vi "Save.vi"(8 "error in (no error)":errorcluster, 10 "Control path":path, 11 "ctl in":refnum<class "ctl.lvclass">) -> (0 "error out":errorcluster, 3 "ctl out":refnum<class "ctl.lvclass">)   [LabVIEW 2012, in "ctl.lvclass"]
uses:
  ctl.lvclass
  ctl.lvclass/ctl.ctl
  _ResManager_v86/IDCloneResMgr.lvlib
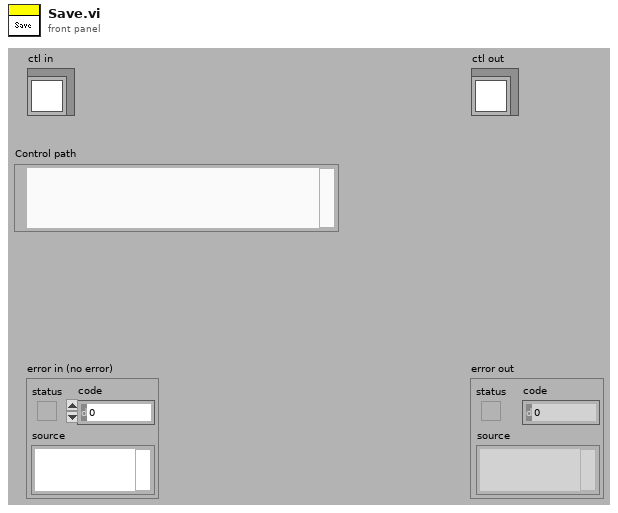
[diagram p1: front panel]
types:
  T1 = cluster{"type":u32, "id":i32, "name":string, "binary data":string}[]
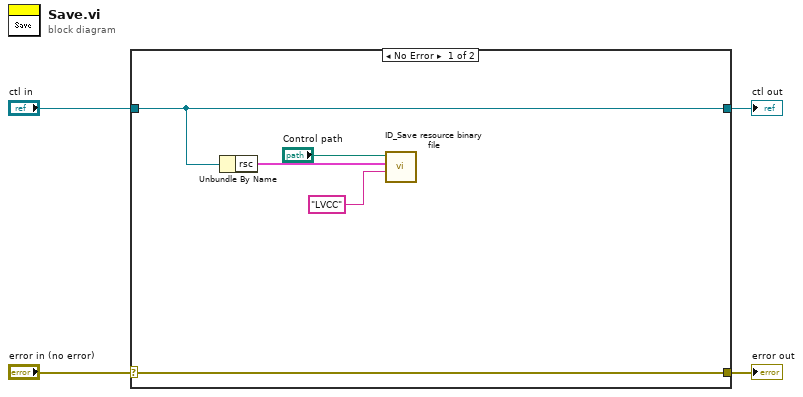
[diagram p0: block diagram]
diagram:
  n1 = case shown="No Error" "error in (no error)" {
    selector: "error in (no error)" -> [w9 w11]
    tunnel: [w9 w11] -> w3
    tunnel: [w8 w10] -> w1
    tunnel: "ctl in" -> [w8 w10]
    frame No Error {
      n2 = Unbundle By Name(w8) -> ("rsc"=w7:T1)
      n3 = call "ID_Save resource binary file.vi"("file type"="LVCC", "resources"=w7, "resource binary file"="Control path") -> ()  [unwired: 9 out]
    }
    frame Error {
    }
  }
  "error out" <- w3
  "ctl out" <- w1
